vi "Is From Actor.vi"(11 "Base Sender in":refnum<class "Base Sender.lvclass">) -> (2 "Is From Actor":bool)   [LabVIEW 2021, in "jettl.lvlib" / "Sender.lvlib" / "Base Sender.lvclass"]
uses:
  Base Sender.lvclass
  Base Sender.lvclass/Base Sender.ctl
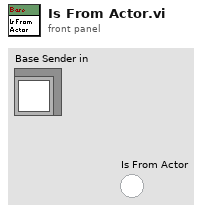
[diagram p1: front panel]
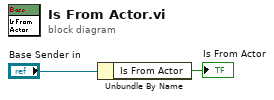
[diagram p0: block diagram]
diagram:
  n1 = Unbundle By Name("Base Sender in") -> ("Is From Actor"=→"Is From Actor":bool)
